vi "IntakeBegin.vi"(8 "error in (no error)":errorcluster) -> (0 "error out":errorcluster)   [LabVIEW 2023]
uses:
  <vilib>/Rock Robotics/SystemInterfaces/DIO/FPGA_DIOChannel.ctl
  <vilib>/Rock Robotics/WPI/ThirdParty/REV Robotics/REVLib/Typedef/Spark MAX Idle Mode.ctl
  <vilib>/Rock Robotics/WPI/Switch/WPI_SwitchOpenLimit.vi
  <vilib>/Rock Robotics/WPI/ThirdParty/REV Robotics/REVLib/SubVI/Public/SPARK Open Brushless.vi
  <vilib>/Rock Robotics/WPI/ThirdParty/REV Robotics/REVLib/SubVI/Public/SPARK Configure Basic Idle Mode.vi
  <vilib>/Rock Robotics/WPI/ThirdParty/REV Robotics/REVLib/SubVI/Public/SPARK Configure Power Smart Current Limit.vi
  <vilib>/Rock Robotics/WPI/ThirdParty/REV Robotics/REVLib/SubVI/Public/SPARK Configure Basic Ramp Rate.vi
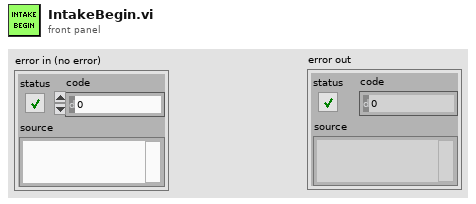
[diagram p1: front panel]
types:
  T1 = typedef "FPGA_DIOChannel.ctl" = enum8{"DIO 0", "DIO 1", "DIO 2", "DIO 3", "DIO 4", "DIO 5", "DIO 6", "DIO 7", "DIO 8", "DIO 9", "DIO MXP 0", "DIO MXP 1", "DIO MXP 2", "DIO MXP 3", "DIO MXP 4", "DIO MXP 5", "DIO MXP 6", "DIO MXP 7", "DIO MXP 8", "DIO MXP 9", "DIO MXP 10", "DIO MXP 11", "DIO MXP 12", "DIO MXP 13", "DIO MXP 14", "DIO MXP 15", "SPI Port CS1", "SPI Port CS2", "SPI Port CS3", "SPI Port MISO", "SPI Port MOSI", "Invalid"}
  T2 = typedef "Spark MAX Idle Mode.ctl" = enum16{"Coast", "Brake"}
  T3 = typedef "WPI_MotorControlDeviceRef.ctl" = cluster{"DeviceStatus":errorcluster, "Type":T4, "PWM":cluster{"PWM Channel":T5, "DeadBand":T6}, "CAN":cluster{"Device Number":u8, "SetOutput VI Ref":variant, "GetOutput VI Ref":variant, "Enable VI Ref":variant, "Disable VI Ref":variant, "Data":variant}, "Invert":bool, "DIO PWM":cluster{"PWM \"Enable\" Channel":T5, "DIOChannel":T1, "PWM Rate":dbl}}
  T4 = typedef "WPI_MotorControlType.ctl" = enum16{"PWM", "CAN", "DIO PWM"}
  T5 = typedef "FPGA_DIOPWMChannel.ctl" = enum8{"PWM 0", "PWM 1", "PWM 2", "PWM 3", "PWM 4", "PWM 5", "PWM 6", "PWM 7", "PWM 8", "PWM 9", "PWM MXP 0", "PWM MXP 1", "PWM MXP 2", "PWM MXP 3", "PWM MXP 4", "PWM MXP 5", "PWM MXP 6", "PWM MXP 7", "PWM MXP 8", "PWM MXP 9", "Invalid"}
  T6 = typedef "WPI_PWMDeadband.ctl" = cluster{"Name":string, "maxPositivePwm":i32, "minPositivePwm":i32, "centerPwm":i32, "maxNegativePwm":i32, "minNegativePwm":i32, "angularRange":u16}
  T7 = typedef "WPI_SwitchDevRef.ctl" = cluster{"DevStatus":errorcluster, "DIO Channel":T1, "CntIndex":T8, "Normally Closed":bool}
  T8 = typedef "FPGA_CounterCtrSystemIndex.ctl" = enum8{"Ctr 0", "Ctr 1", "Ctr 2", "Ctr 3", "Ctr 4", "Ctr 5", "Ctr 6", "Ctr 7", "Invalid"}
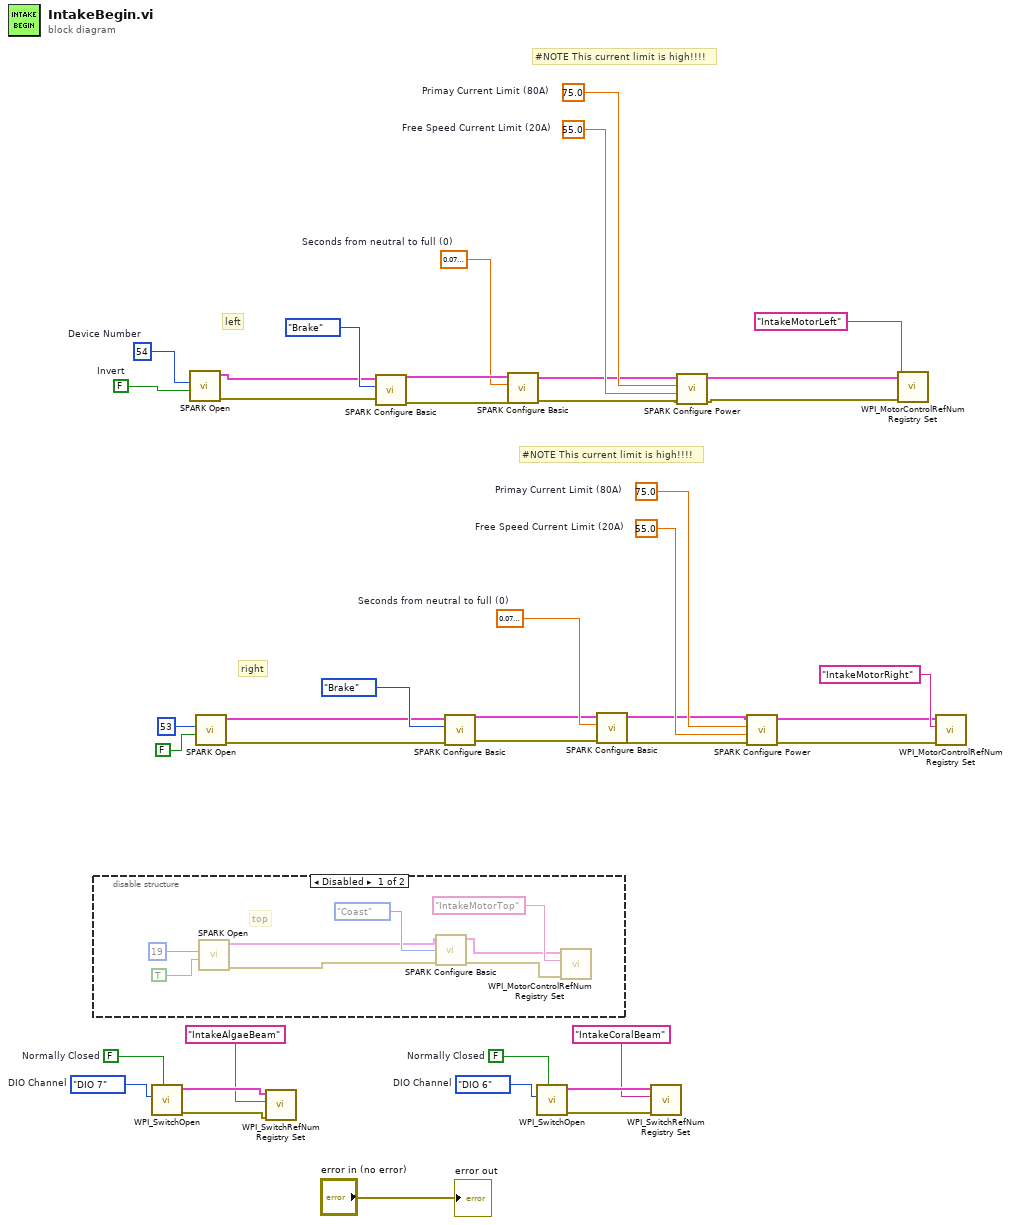
[diagram p0: block diagram]
diagram:
  w5 = sgl 0.08  # Seconds from neutral to full (0)
  w6 = sgl 0.08  # Seconds from neutral to full (0)
  w13 = 55.0  # Free Speed Current Limit (20A)
  w14 = 75.0  # Primay Current Limit (80A)
  w17 = 55.0  # Free Speed Current Limit (20A)
  w18 = 75.0  # Primay Current Limit (80A)
  w22 = FALSE  # Normally Closed
  w23 = FPGA_DIOChannel."DIO 6"  # DIO Channel
  w28 = FALSE  # Normally Closed
  w29 = FPGA_DIOChannel."DIO 7"  # DIO Channel
  w40 = FALSE  # Invert
  w41 = u8 54  # Device Number
  # "#NOTE This current limit is high!!!!"
  # "#NOTE This current limit is high!!!!"
  # "right"
  # "left"
  n1 = disable-structure shown="Disabled" {
    frame Disabled {
      # "top"
      n2 = call-poly <vilib>:"SPARK Open.vi"("Invert"=TRUE, "Device Number"=u8 19) -> ("error out"=w45:errorcluster, "MotorControlDeviceRef"=w46:T3)  [unwired: 8 in]
      n3 = call-poly <vilib>:"SPARK Configure Basic.vi"("error in (no error)"=w45, "Idle Mode"=Spark_MAX_Idle_Mode."Coast", "MotorControlDeviceRef in"=w46) -> ("error out"=w42:errorcluster, "MotorControlDeviceRef out"=w43:T3)  [unwired: 7 in]
      n4 = call <vilib>:"WPI_MotorControlRefNum Registry Set.vi"("error in (no error)"=w42, "refnum name"="IntakeMotorTop", "MotorControlDevRef"=w43) -> ()  [unwired: 7 in, 2 out]
    }
    frame Enabled {
    }
  }
  n5 = call-poly <vilib>:"WPI_SwitchOpen.vi"("Normally Closed"=w28, "DIO Channel"=w29) -> ("error out"=w26:errorcluster, "SwitchDevRef"=w27:T7)  [unwired: 8 in]
  n6 = call-poly <vilib>:"SPARK Open.vi"("Invert"=w40, "Device Number"=w41) -> ("error out"=w32:errorcluster, "MotorControlDeviceRef"=w33:T3)  [unwired: 8 in]
  n7 = call-poly <vilib>:"SPARK Open.vi"("Invert"=FALSE, "Device Number"=u8 53) -> ("error out"=w35:errorcluster, "MotorControlDeviceRef"=w34:T3)  [unwired: 8 in]
  n8 = call <vilib>:"WPI_SwitchRefNum Registry Set.vi"("error in (no error)"=w26, "refnum name"="IntakeAlgaeBeam", "SwitchDevRef"=w27) -> ()  [unwired: 7 in, 2 out]
  n9 = call-poly <vilib>:"SPARK Configure Basic.vi"("error in (no error)"=w32, "Idle Mode"=Spark_MAX_Idle_Mode."Brake", "MotorControlDeviceRef in"=w33) -> ("error out"=w9:errorcluster, "MotorControlDeviceRef out"=w10:T3)  [unwired: 7 in]
  n10 = call-poly <vilib>:"SPARK Configure Basic.vi"("error in (no error)"=w35, "Idle Mode"=Spark_MAX_Idle_Mode."Brake", "MotorControlDeviceRef in"=w34) -> ("error out"=w3:errorcluster, "MotorControlDeviceRef out"=w4:T3)  [unwired: 7 in]
  n11 = call-poly <vilib>:"SPARK Configure Basic.vi"("error in (no error)"=w9, "Seconds from neutral to full (0)"=w6, "MotorControlDeviceRef in"=w10) -> ("error out"=w8:errorcluster, "MotorControlDeviceRef"=w7:T3)  [unwired: 7 in]
  n12 = call-poly <vilib>:"WPI_SwitchOpen.vi"("Normally Closed"=w22, "DIO Channel"=w23) -> ("error out"=w20:errorcluster, "SwitchDevRef"=w21:T7)  [unwired: 8 in]
  n13 = call-poly <vilib>:"SPARK Configure Basic.vi"("error in (no error)"=w3, "Seconds from neutral to full (0)"=w5, "MotorControlDeviceRef in"=w4) -> ("error out"=w1:errorcluster, "MotorControlDeviceRef"=w2:T3)  [unwired: 7 in]
  n14 = call <vilib>:"WPI_SwitchRefNum Registry Set.vi"("error in (no error)"=w20, "refnum name"="IntakeCoralBeam", "SwitchDevRef"=w21) -> ()  [unwired: 7 in, 2 out]
  n15 = call-poly <vilib>:"SPARK Configure Power.vi"("error in (no error)"=w8, "Free Speed Current Limit (20A)"=w17, "Primay Current Limit (80A)"=w18, "MotorControlDeviceRef in"=w7) -> ("error out"=w15:errorcluster, "MotorControlDeviceRef out"=w16:T3)  [unwired: 6 in]
  n16 = call-poly <vilib>:"SPARK Configure Power.vi"("error in (no error)"=w1, "Free Speed Current Limit (20A)"=w13, "Primay Current Limit (80A)"=w14, "MotorControlDeviceRef in"=w2) -> ("error out"=w11:errorcluster, "MotorControlDeviceRef out"=w12:T3)  [unwired: 6 in]
  n17 = call <vilib>:"WPI_MotorControlRefNum Registry Set.vi"("error in (no error)"=w15, "refnum name"="IntakeMotorLeft", "MotorControlDevRef"=w16) -> ()  [unwired: 7 in, 2 out]
  n18 = call <vilib>:"WPI_MotorControlRefNum Registry Set.vi"("error in (no error)"=w11, "refnum name"="IntakeMotorRight", "MotorControlDevRef"=w12) -> ()  [unwired: 7 in, 2 out]
  "error out" <- "error in (no error)"
